vi "2 GrabCurrentWaypoint.vi"() -> (2 "Current Waypoint":refnum<class "Waypoint.lvclass">)   [LabVIEW 2011]
doc: "Returns the current waypoint, using the Global waypoints array and the current waypoint index."
uses:
  2 Classes/Waypoint/Waypoint.lvclass
  2 Globals/2 Global.vi
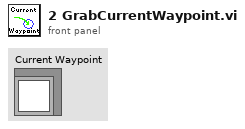
[diagram p1: front panel]
types:
  T1 = typedef "Current Waypoint.ctl" = i32
  T2 = typedef "Waypoints List.ctl" = refnum<class "Waypoint.lvclass">[]
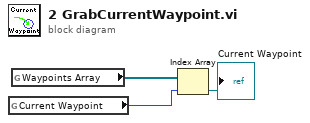
[diagram p0: block diagram]
diagram:
  n1 = global read "2 Global.vi" "Current Waypoint"() -> (w2:T1)
  n2 = global read "2 Global.vi" "Waypoints Array"() -> (w3:T2)
  n3 = Index Array(array=w3, index=w2) -> (element=→"Current Waypoint":refnum<class "Waypoint.lvclass">)
